vi "Vibration.vi"() -> ()   [LabVIEW 2012]
uses:
  <vilib>/Analysis/NI_AALPro.lvlib
panel:
  out "选项卡":T1(tab)
  in  "装置IP":string
  in  "?":bool
  in  "灵敏度4(mv/g)":i32=1 min=1
  in  "灵敏度3(mv/g)":i32=1 min=1
  in  "灵敏度2(mv/g)":i32=1 min=1
  in  "采样率4(ksps)":T2(ring)=enum."105.468"
  in  "采样率3(ksps)":T2(ring)=enum."105.468"
  in  "采样率2(ksps)":T2(ring)=enum."105.468"
  in  "灵敏度1(mv/g)":i32=1 min=1
  in  "采样率1(ksps)":T2(ring)=enum."105.468"
  in  "?":bool
  in  "?":bool
  in  "开始":bool
  in  "?":bool
  in  "设置装置网关":string
  in  "设置装置子网掩码":string
  in  "设置装置IP":string
  in  "?":bool
  in  "是否开启电流源":u8(knob)=1 scale=0.0..1.0
  in  "是否进行自校准":u8(knob) scale=0.0..1.0
  in  "?":bool
  in  "?":path
  in  "是否保存数据":u8(knob) scale=0.0..1.0
  in  "?":bool
  out "进度条":dbl(slide) scale=0.0..99.0
  out "字符串":string
  out "波形卡":enum32{"波形卡 1", "波形卡 2", "波形卡 3"}(tab)
  in  "AC/DC":bool
  in  "Y轴调整":dbl(knob)=5.0 min=0.0001 max=5.0 step=0.001 scale=0.0001..5.0
  out "?":dbl[][](graph)
  out "?":dbl[][](graph)
  in  "X轴调整":u32(knob)=50000 min=1000 max=50000 step=100 scale=1100.0..50000.0
  in  "通道1":bool=TRUE
  in  "通道2":bool=TRUE
  in  "通道3":bool=TRUE
  in  "通道4":bool=TRUE
  out "?":u16[](graph)
  out "转 \n速":u16(knob) scale=0.0..20000.0
  # "PageUp\nPageDown\n微调"
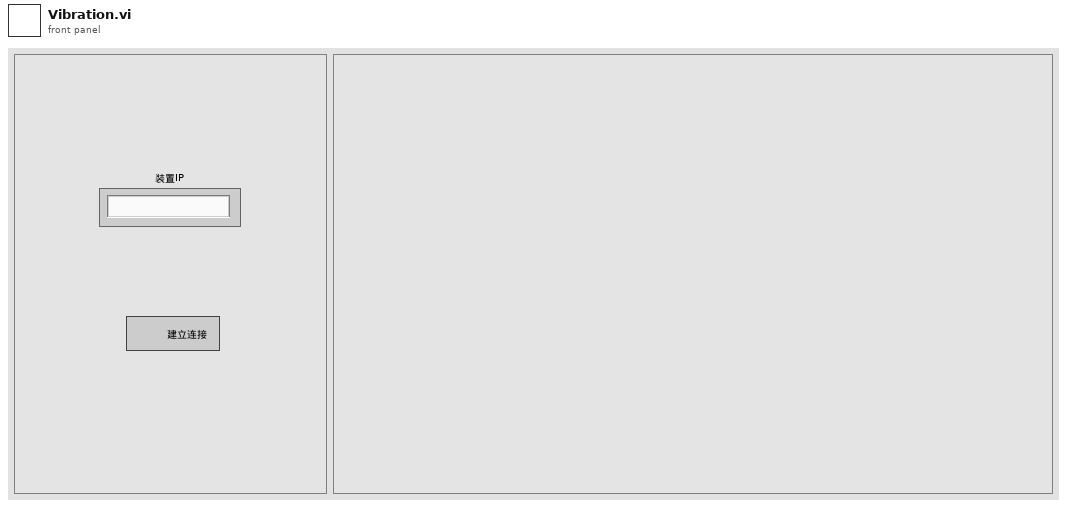
[diagram p1: front panel]
types:
  T1 = enum32{"选项卡 1", "选项卡 2", "选项卡 3", "选项卡 4", "选项卡 5", "选项卡 6", "选项卡 7"}
  T2 = enum16{"", "105.468", "52.734", "35.156", "26.367", "21.094", "17.578", "15.067", "13.184", "11.719", "10.545"}
  T3 = enum8{"Enabled", "Disabled", "Disabled and Grayed Out"}
  T4 = cluster{"SavePath":path, "SAVE?":bool, "connection ID":refnum<k5>}
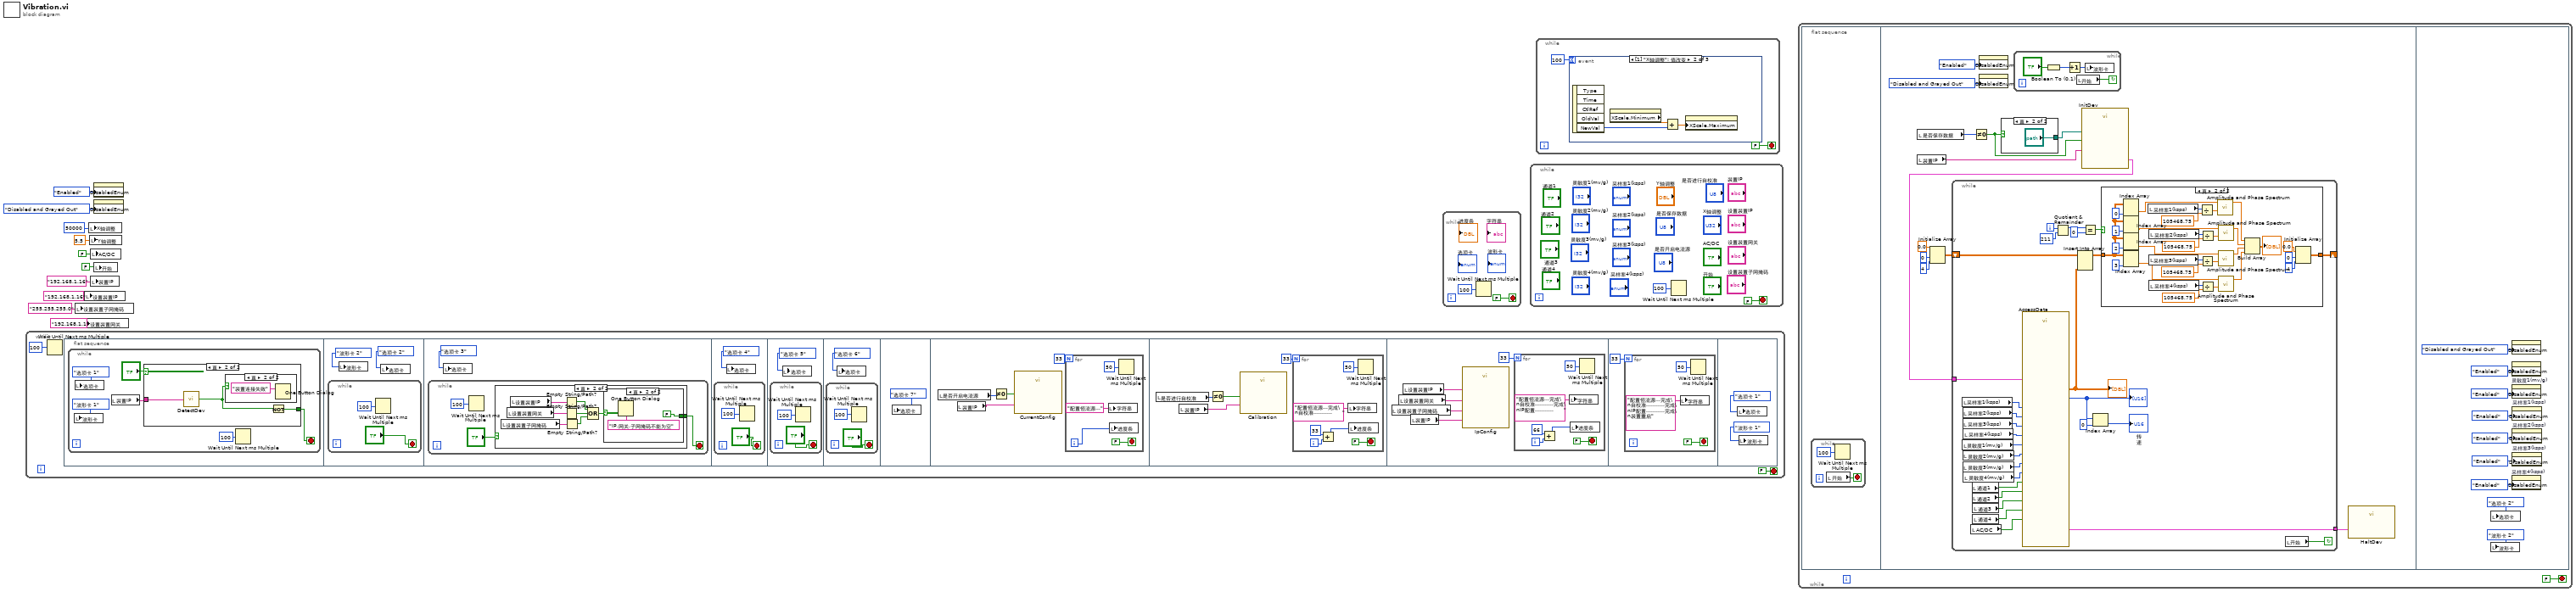
[diagram p0: block diagram]
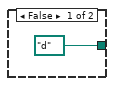
[diagram p3: hidden frame]
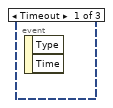
[diagram p4: hidden frame]
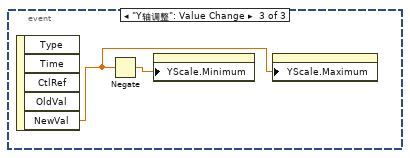
[diagram p5: hidden frame]
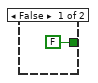
[diagram p6: hidden frame]
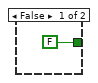
[diagram p8: hidden frame]
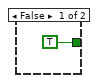
[diagram p9: hidden frame]
diagram:
  n1 = while {
    stop <- FALSE stop-if-true
    n2 = Wait Until Next ms Multiple(millisecond multiple=u32 100 ("毫秒倍数")) -> ()  [unwired: 1 out]
    n3 = flat-sequence {
      frame #0 {
        n4 = while {
          stop <- w17 stop-if-true
          n5 = local write "波形卡"(enum32{"波形卡 1", "波形卡 2", "波形卡 3"}."波形卡 1" ("波形卡")) -> ()
          n6 = local write "选项卡"(T1."选项卡 1" ("选项卡")) -> ()
          n7 = local read "装置IP"() -> (w13:string)
          n8 = case shown="真" "?" {
            tunnel: [FALSE w22] -> w17
            tunnel: w13 -> [_ w20]
            frame False {
            }
            frame True {
              n9 = call "DetectDev.vi"("IP."=w20) -> ("Fail"=w21:bool)
              n10 = case shown="真" w21 {
                frame False {
                }
                frame True {
                  n11 = One Button Dialog(message="装置连接失败" ("消息")) -> ()  [unwired: 1 in, 1 out]
                }
              }
              n12 = Not(x=w21) -> (.not. x?=w22:bool)
            }
          }
          n13 = Wait Until Next ms Multiple(millisecond multiple=u32 100 ("毫秒倍数")) -> ()  [unwired: 1 out]
        }
      }
      frame #1 {
        n14 = while {
          stop <- "?" stop-if-true
          n15 = Wait Until Next ms Multiple(millisecond multiple=u32 100 ("毫秒倍数")) -> ()  [unwired: 1 out]
        }
        n16 = local write "波形卡"(enum32{"波形卡 1", "波形卡 2", "波形卡 3"}."波形卡 2" ("波形卡")) -> ()
        n17 = local write "选项卡"(T1."选项卡 2" ("选项卡")) -> ()
      }
      frame #2 {
        n18 = while {
          stop <- w29 stop-if-true
          n19 = Wait Until Next ms Multiple(millisecond multiple=u32 100 ("毫秒倍数")) -> ()  [unwired: 1 out]
          n20 = case shown="真" "?" {
            tunnel: [FALSE w33] -> w29
            frame False {
            }
            frame True {
              n21 = local read "设置装置子网掩码"() -> (w40:string)
              n22 = local read "设置装置网关"() -> (w39:string)
              n23 = local read "设置装置IP"() -> (w38:string)
              n24 = Empty String/Path?(string/path=w38) -> (empty?=w35:bool)
              n25 = Empty String/Path?(string/path=w39) -> (empty?=w36:bool)
              n26 = Empty String/Path?(string/path=w40) -> (empty?=w37:bool)
              n27 = Compound Arithmetic op=OR(w35, w36, w37) -> (w34:bool)
              n28 = case shown="真" w34 {
                tunnel: [TRUE FALSE] -> w33
                frame False {
                }
                frame True {
                  n29 = One Button Dialog(message="IP,网关,子网掩码不能为空" ("消息")) -> ()  [unwired: 1 in, 1 out]
                }
              }
            }
          }
        }
        n30 = local write "选项卡"(T1."选项卡 3" ("选项卡")) -> ()
      }
      frame #3 {
        n31 = while {
          stop <- "?" stop-if-true
          n32 = Wait Until Next ms Multiple(millisecond multiple=u32 100 ("毫秒倍数")) -> ()  [unwired: 1 out]
        }
        n33 = local write "选项卡"(T1."选项卡 4" ("选项卡")) -> ()
      }
      frame #4 {
        n34 = while {
          stop <- "?" stop-if-true
          n35 = Wait Until Next ms Multiple(millisecond multiple=u32 100 ("毫秒倍数")) -> ()  [unwired: 1 out]
        }
        n36 = local write "选项卡"(T1."选项卡 5" ("选项卡")) -> ()
      }
      frame #5 {
        n37 = while {
          stop <- "?" stop-if-true
          n38 = Wait Until Next ms Multiple(millisecond multiple=u32 100 ("毫秒倍数")) -> ()  [unwired: 1 out]
        }
        n39 = local write "选项卡"(T1."选项卡 6" ("选项卡")) -> ()
      }
      frame #6 {
        n40 = local write "选项卡"(T1."选项卡 7" ("选项卡")) -> ()
      }
      frame #7 {
        n41 = local read "是否开启电流源"() -> (w55:u8)
        n42 = local read "装置IP"() -> (w54:string)
        n43 = Not Equal To 0?(x=w55) -> (x != 0?=w56:bool)
        n44 = call "CurrentConfig.vi"("Current"=w56, "IP"=w54) -> ()
        n45 = for {
          N: 33 -> [_]
          i -> [w58]
          stop <- FALSE stop-if-true
          n46 = local write "字符串"("配置恒流源..." ("字符串")) -> ()
          n47 = local write "进度条"(w58) -> ()
          n48 = Wait Until Next ms Multiple(millisecond multiple=u32 50 ("毫秒倍数")) -> ()  [unwired: 1 out]
        }
      }
      frame #8 {
        n49 = local read "是否进行自校准"() -> (w63:u8)
        n50 = local read "装置IP"() -> (w62:string)
        n51 = Not Equal To 0?(x=w63) -> (x != 0?=w64:bool)
        n52 = call "Calibration.vi"("Enable"=w64, "IP."=w62) -> ()
        n53 = for {
          N: 33 -> [_]
          i -> [w68]
          stop <- FALSE stop-if-true
          n54 = Add(x=33, y=w68) -> (x+y=w67:i32)
          n55 = local write "字符串"("配置恒流源...完成\n自校准...........      " ("字符串")) -> ()
          n56 = local write "进度条"(w67) -> ()
          n57 = Wait Until Next ms Multiple(millisecond multiple=u32 50 ("毫秒倍数")) -> ()  [unwired: 1 out]
        }
      }
      frame #9 {
        n58 = local read "设置装置子网掩码"() -> (w74:string)
        n59 = local read "设置装置网关"() -> (w73:string)
        n60 = local read "设置装置IP"() -> (w72:string)
        n61 = local read "装置IP"() -> (w75:string)
        n62 = call "IpConfig.vi"("Gateway"=w73, "SubnetMask"=w74, "IP"=w72, "CurrentIP"=w75) -> ()
        n63 = for {
          N: 33 -> [_]
          i -> [w79]
          stop <- FALSE stop-if-true
          n64 = Add(x=66, y=w79) -> (x+y=w78:i32)
          n65 = local write "字符串"("配置恒流源...完成\n自校准...........完成\nIP配置...........      " ("字符串")) -> ()
          n66 = local write "进度条"(w78) -> ()
          n67 = Wait Until Next ms Multiple(millisecond multiple=u32 50 ("毫秒倍数")) -> ()  [unwired: 1 out]
        }
      }
      frame #10 {
        n68 = for {
          N: 33 -> [_]
          stop <- FALSE stop-if-true
          n69 = local write "字符串"("配置恒流源...完成\n自校准...........完成\nIP配置...........完成\n装置重启" ("字符串")) -> ()
          n70 = Wait Until Next ms Multiple(millisecond multiple=u32 50 ("毫秒倍数")) -> ()  [unwired: 1 out]
        }
      }
      frame #11 {
        n71 = local write "选项卡"(T1."选项卡 1" ("选项卡")) -> ()
        n72 = local write "波形卡"(enum32{"波形卡 1", "波形卡 2", "波形卡 3"}."波形卡 1" ("波形卡")) -> ()
      }
    }
  }
  n73 = local write "设置装置子网掩码"("255.255.255.0" ("新子网掩码")) -> ()
  n74 = local write "设置装置网关"("192.168.1.1" ("新网关")) -> ()
  n75 = local write "设置装置IP"("192.168.1.16" ("新装置IP")) -> ()
  n76 = local write "X轴调整"(u16 50000 ("X轴调整")) -> ()
  n77 = local write "Y轴调整"(5.5 ("Y轴调整")) -> ()
  n78 = local write "AC/DC"(FALSE ("AC/DC")) -> ()
  n79 = local write "装置IP"("192.168.1.16" ("装置IP")) -> ()
  n80 = property class="Bool"("DisabledEnum"=T3."Enabled" ("禁用")) -> ()  [unwired: 2 in, 2 out]
  n81 = property class="Bool (严格)"("DisabledEnum"=T3."Disabled and Grayed Out" ("禁用")) -> ()  [unwired: 2 in, 2 out]
  n82 = local write "开始"(FALSE ("开始")) -> ()
  n83 = while {
    stop <- FALSE stop-if-true
    n84 = Wait Until Next ms Multiple(millisecond multiple=u32 100 ("毫秒倍数")) -> ()  [unwired: 1 out]
  }
  n85 = while {
    stop <- FALSE stop-if-true
    n86 = Wait Until Next ms Multiple(millisecond multiple=u32 100 ("毫秒倍数")) -> ()  [unwired: 1 out]
  }
  n87 = while {
    stop <- FALSE stop-if-true
    n88 = event shown="[1] \"X轴调整\": 值改变" {
      selector: _ -> [_ _ _]
      dyn-events: _ -> [_ _ _]
      timeout: 100 -> [_ _ _]
      event Timeout {
        n89 = event-data() -> ()  [unwired: 1 in, 2 out]
      }
      event "X轴调整": Value Change {
        n90 = event-data() -> ("NewVal"=w97:u32)  [unwired: 1 in, 4 out]
        n91 = property class="WFChart (严格)"() -> ("XScale.Minimum"=w96:dbl)  [unwired: 2 in, 2 out]
        n92 = Add(x=w96, y=w97) -> (x+y=w95:dbl)
        n93 = property class="WFChart (严格)"("XScale.Maximum"=w95) -> ()  [unwired: 2 in, 2 out]
      }
      event "Y轴调整": Value Change {
        n94 = event-data() -> ("NewVal"=w98:dbl)  [unwired: 1 in, 4 out]
        n95 = Negate(x=w98) -> (-x=w99:dbl)
        n96 = property class="WFChart (严格)"("YScale.Minimum"=w99) -> ()  [unwired: 2 in, 2 out]
        n97 = property class="WFChart (严格)"("YScale.Maximum"=w98) -> ()  [unwired: 2 in, 2 out]
      }
    }
  }
  n98 = while {
    stop <- FALSE stop-if-true
    n99 = flat-sequence {
      frame #0 {
        n100 = while {
          stop <- w101 stop-if-true
          n101 = local read "开始"() -> (w101:bool)
          n102 = Wait Until Next ms Multiple(millisecond multiple=u32 100 ("毫秒倍数")) -> ()  [unwired: 1 out]
        }
      }
      frame #1 {
        n103 = local read "是否保存数据"() -> (w114:u8)
        n104 = local read "装置IP"() -> (w109:string)
        n105 = Initialize Array(0.0 ("元素"), 0 ("维数大小"), 4 ("维数大小")) -> (w103:dbl[][])
        n106 = Not Equal To 0?(x=w114) -> (x != 0?=w110:bool)
        n107 = property class="Bool (严格)"("DisabledEnum"=T3."Enabled" ("禁用")) -> ()  [unwired: 2 in, 2 out]
        n108 = property class="Bool"("DisabledEnum"=T3."Disabled and Grayed Out" ("禁用")) -> ()  [unwired: 2 in, 2 out]
        n109 = case shown="真" w110 {
          tunnel: [path "d:/" ("路径（使用对话框）") "?"] -> w111
          frame False {
          }
          frame True {
          }
        }
        n110 = while {
          stop <- w174 continue-if-true
          n111 = Boolean To (0,1)(Boolean="?") -> (0, 1=w177:i16)
          n112 = Increment(x=w177) -> (x+1=w175:i16)
          n113 = local read "开始"() -> (w174:bool)
          n114 = local write "波形卡"(w175) -> ()
        }
        n115 = call "InitDev.vi"("SAVE?"=w110, "IP地址"=w109, "SavePath"=w111) -> ("输出簇"=w108:T4)
        n116 = while {
          tunnel: w108 -> [w139]
          tunnel: [w138] -> w107
          shift-right: [w121] -> _
          shift-left: w103 -> [w123]
          i -> [w118]
          stop <- w140 continue-if-true
          n117 = local read "采样率1(ksps)"() -> (w137:T2)
          n118 = local read "灵敏度1(mv/g)"() -> (w133:i32)
          n119 = local read "采样率2(ksps)"() -> (w136:T2)
          n120 = local read "采样率3(ksps)"() -> (w135:T2)
          n121 = local read "灵敏度2(mv/g)"() -> (w131:i32)
          n122 = local read "灵敏度3(mv/g)"() -> (w130:i32)
          n123 = local read "采样率4(ksps)"() -> (w134:T2)
          n124 = local read "灵敏度4(mv/g)"() -> (w129:i32)
          n125 = local read "AC/DC"() -> (w124:bool)
          n126 = local read "通道1"() -> (w128:bool)
          n127 = local read "通道2"() -> (w127:bool)
          n128 = local read "通道3"() -> (w126:bool)
          n129 = local read "通道4"() -> (w125:bool)
          n130 = call "AccessData.vi"("Sensitivity1"=w133, "Sensitivity2"=w131, "Sensitivity3"=w130, "Sensitivity4"=w129, "输入簇"=w139, "CH1Enable"=w128, "CH2Enable"=w127, "CH3Enable"=w126, "CH4Enable"=w125, "RmOffset"=w124, "SamplRate1"=w137, "SamplRate2"=w136, "SamplRate3"=w135, "SamplRate4"=w134) -> ("VibrationWave"=w116:dbl[][], "Speed"=w132:u16[], "输出簇"=w138:T4)  [unwired: 2 in, 1 out]
          "?" <- w116
          "?" <- w132
          n131 = Quotient & Remainder(x=w118, y=u8 211 ("x")) -> (x-y*floor(x/y)=w120:i32)  [unwired: 1 out]
          n132 = Insert Into Array(array=w123, new element=w116) -> (w122:dbl[][])  [unwired: 2 in]
          n133 = Equal?(x=w120, y=0) -> (x = y?=w117:bool)
          n134 = Index Array(array=w132, index=0 ("索引")) -> (element=→"转 \n速":u16)
          n135 = case shown="真" w117 {
            tunnel: w122 -> [w143 w148]
            tunnel: [w143 w144] -> w121
            frame False {
            }
            frame True {
              n136 = Index Array(array=w148, index (col)=0 ("禁用的索引 (列)")) -> (element=w150:dbl[])  [unwired: 1 in]
              n137 = Index Array(array=w148, index (col)=1 ("禁用的索引 (列)")) -> (element=w157:dbl[])  [unwired: 1 in]
              n138 = Index Array(array=w148, index (col)=2 ("禁用的索引 (列)")) -> (element=w156:dbl[])  [unwired: 1 in]
              n139 = Index Array(array=w148, index (col)=3 ("禁用的索引 (列)")) -> (element=w155:dbl[])  [unwired: 1 in]
              n140 = local read "采样率1(ksps)"() -> (w167:T2)
              n141 = local read "采样率3(ksps)"() -> (w161:T2)
              n142 = local read "采样率2(ksps)"() -> (w164:T2)
              n143 = local read "采样率4(ksps)"() -> (w158:T2)
              n144 = Divide(x=w167, y=105468.75 ("dt")) -> (x/y=w168:dbl)
              n145 = Divide(x=w161, y=105468.75 ("dt")) -> (x/y=w162:dbl)
              n146 = Divide(x=w164, y=105468.75 ("dt")) -> (x/y=w165:dbl)
              n147 = Divide(x=w158, y=105468.75 ("dt")) -> (x/y=w159:dbl)
              n148 = call <vilib>:"Amplitude and Phase Spectrum.vi"("dt"=w168, "Signal (V)"=w150) -> ("Amp Spectrum Mag (Vrms)"=w154:dbl[])  [unwired: 1 in, 2 out]
              n149 = call <vilib>:"Amplitude and Phase Spectrum.vi"("dt"=w162, "Signal (V)"=w156) -> ("Amp Spectrum Mag (Vrms)"=w151:dbl[])  [unwired: 1 in, 2 out]
              n150 = call <vilib>:"Amplitude and Phase Spectrum.vi"("dt"=w165, "Signal (V)"=w157) -> ("Amp Spectrum Mag (Vrms)"=w153:dbl[])  [unwired: 1 in, 2 out]
              n151 = call <vilib>:"Amplitude and Phase Spectrum.vi"("dt"=w159, "Signal (V)"=w155) -> ("Amp Spectrum Mag (Vrms)"=w152:dbl[])  [unwired: 1 in, 2 out]
              n152 = Build Array(w154, w153, w151, w152) -> (→"?":dbl[][])
              n153 = Initialize Array(0.0 ("元素"), 0 ("维数大小"), 4 ("维数大小")) -> (w144:dbl[][])
            }
          }
          n154 = local read "开始"() -> (w140:bool)
        }
        n155 = call "HaltDev.vi"("输入簇"=w107) -> ()
      }
      frame #2 {
        n156 = local write "波形卡"(enum32{"波形卡 1", "波形卡 2", "波形卡 3"}."波形卡 2" ("波形卡")) -> ()
        n157 = local write "选项卡"(T1."选项卡 2" ("选项卡")) -> ()
        n158 = property class="Bool (严格)"("DisabledEnum"=T3."Disabled and Grayed Out" ("禁用")) -> ()  [unwired: 2 in, 2 out]
        n159 = property class="Bool"("DisabledEnum"=T3."Enabled" ("禁用")) -> ()  [unwired: 2 in, 2 out]
        n160 = property on="灵敏度1(mv/g)" class="DigNum (严格)"("DisabledEnum"=T3."Enabled" ("禁用")) -> ()  [unwired: 2 in, 2 out]
        n161 = property on="采样率4(ksps)" class="Enum (严格)"("DisabledEnum"=T3."Enabled" ("禁用")) -> ()  [unwired: 2 in, 2 out]
        n162 = property on="采样率1(ksps)" class="Enum (严格)"("DisabledEnum"=T3."Enabled" ("禁用")) -> ()  [unwired: 2 in, 2 out]
        n163 = property on="采样率2(ksps)" class="Enum (严格)"("DisabledEnum"=T3."Enabled" ("禁用")) -> ()  [unwired: 2 in, 2 out]
        n164 = property on="采样率3(ksps)" class="Enum (严格)"("DisabledEnum"=T3."Enabled" ("禁用")) -> ()  [unwired: 2 in, 2 out]
      }
    }
  }
